vi "_save_csv_EVM_EIRP_Selection.vi"(7 "NoteName":string="SingleCh_", 11 "array in":string[][](array[string])) -> (3 "FileName":string)   [LabVIEW 2023]
uses:
  <vilib>/Utility/file.llb/Write Delimited Spreadsheet (string).vi
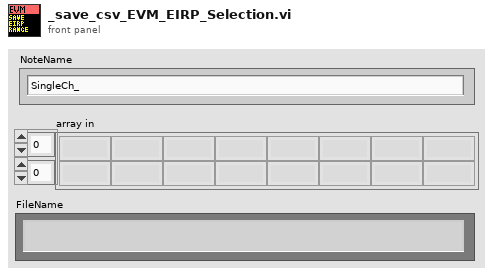
[diagram p1: front panel]
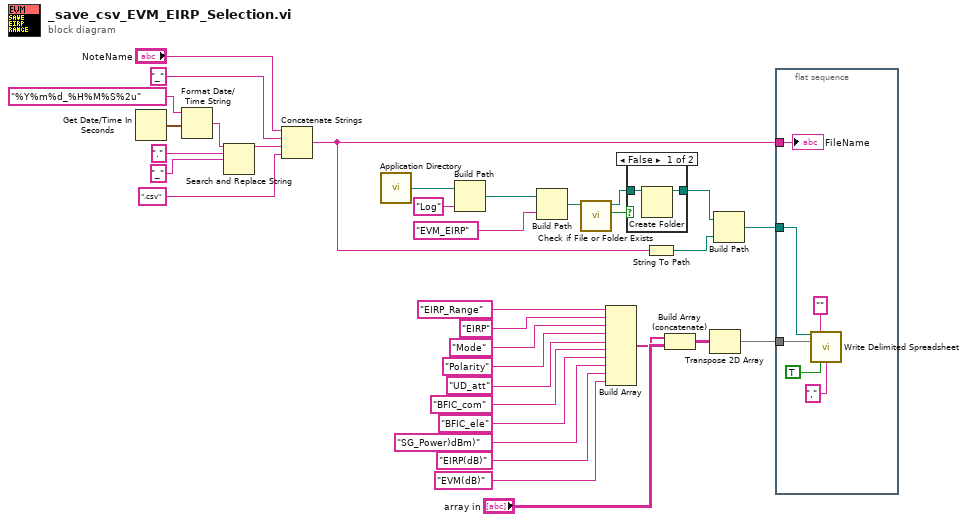
[diagram p0: block diagram]
diagram:
  n1 = Get Date/Time In Seconds() -> (seconds since 1Jan1904=w14:timestamp)
  n2 = Format Date/Time String(time format string (%c)="%Y%m%d_%H%M%S%2u", seconds (now)=w14) -> (date/time string=w12:string)  [unwired: 1 in]
  n3 = Search and Replace String(input string=w12, search string=".", replace string="_") -> (result string=w9:string)  [unwired: 5 in, 3 out]
  n4 = Concatenate Strings("NoteName", "_", w9, ".csv" ("delimiter (\\t)")) -> (w31:string)
  n5 = call <vilib>:"Application Directory.vi"() -> ("Application Directory"=w6:path)
  n6 = Build Path(base path=w6, name or relative path="Log") -> (appended path=w4:path)
  n7 = Build Path(base path=w4, name or relative path="EVM_EIRP") -> (appended path=w3:path)
  n8 = call <vilib>:"Check if File or Folder Exists.vi"("path"=w3) -> ("file or folder exists?"=w30:bool, "dup path"=w29:path)  [unwired: 8 in, 1 out]
  n9 = Build Array("EIRP_Range", "EIRP", "Mode", "Polarity", "UD_att", "BFIC_com", "BFIC_ele", "SG_Power)dBm)", "EIRP(dB)", "EVM(dB)") -> (w19:string[])
  n10 = case shown="False" w30 {
    tunnel: w29 -> [w36 w37]
    tunnel: [w35 w37] -> w28
    frame False {
      n11 = Create Folder(path (use dialog)=w36) -> (created path=w35:path)  [unwired: 2 in, 2 out]
    }
    frame True {
    }
  }
  n12 = String To Path(string=w31) -> (path=w33:path)
  n13 = Build Array (concatenate)(w19, "array in") -> (w25:string[][])
  n14 = Transpose 2D Array(2D array=w25) -> (transposed array=w27:string[][])
  n15 = Build Path(base path=w28, name or relative path=w33) -> (appended path=w32:path)
  n16 = flat-sequence {
    tunnel: w32 -> [w42]
    tunnel: w31 -> [w40]
    tunnel: w27 -> [w38]
    frame #0 {
      n17 = call-poly <vilib>:"Write Delimited Spreadsheet.vi"("file path (dialog if empty)"=w42, "format (%s)"="" ("format (%.3f)"), "2D data"=w38, "transpose? (no:F)"=TRUE, "delimiter (\\t)"="," ("delimiter (\\t)")) -> ()  [unwired: 9 in, 2 out]
      "FileName" <- w40
    }
  }
